vi "fgv_5413_visa.vi"(7 "cmd":T2, 8 "error in":errorcluster) -> (0 "error out":errorcluster)   [LabVIEW 2021]
uses:
  ctrl/PXIe-5413.ctl
  ctrl/rw.ctl
  <instrlib>/niFgen/niFgen.llb/niFgen Output Mode.ctl
  <instrlib>/niFgen/niFgen.llb/niFgen Create Waveform (DBL).vi
panel:
  out "wfm":dbl[](graph)=[0.0, 0.024541228522912288, 0.049067674327418015, 0.07356456359966743, 0.0980171403295606, 0.1224106751992162, 0.14673047445536175, 0.17096188876030122, 0.19509032201612828, 0.2191012401568698, 0.2429801799032639, 0.26671275747489837, 0.2902846772544624, 0.31368174039889146, 0.33688985339222005, 0.3598950365349881, 0.3826834323650898, 0.40524131400498986, 0.4275550934302821, 0.4496113296546066, 0.47139673682599764, 0.49289819222978404, 0.5141027441932218, 0.5349976198870973, 0.5555702330196023, 0.5758081914178453, 0.5956993044924334, 0.6152315905806269, 0.6343932841636455, 0.6531728429537769, 0.6715589548470184, 0.689540544737067, 0.7071067811865476, 0.724247082951467, 0.7409511253549591, 0.7572088465064847, 0.773010453362737, 0.7883464276266063, 0.8032075314806449, 0.8175848131515838, 0.8314696123025452, 0.8448535652497072, 0.8577286100002721, 0.8700869911087116, 0.881921264348355, 0.8932243011955154, 0.9039892931234433, 0.9142097557035308, 0.9238795325112867, 0.9329927988347391, 0.9415440651830208, 0.9495281805930369, 0.9569403357322089, 0.9637760657954401, 0.9700312531945441, 0.9757021300385287, 0.9807852804032305, 0.9852776423889413, 0.989176509964781, 0.9924795345987101, 0.9951847266721969, 0.9972904566786903, 0.9987954562051724, 0.9996988186962044, 1.0, 0.9996988186962044, 0.9987954562051724, 0.9972904566786903, 0.9951847266721969, 0.9924795345987101, 0.989176509964781, 0.9852776423889413, 0.9807852804032305, 0.9757021300385286, 0.9700312531945441, 0.9637760657954398, 0.9569403357322089, 0.9495281805930367, 0.9415440651830208, 0.9329927988347388, 0.9238795325112867, 0.9142097557035306, 0.9039892931234433, 0.8932243011955152, 0.881921264348355, 0.8700869911087113, 0.8577286100002721, 0.844853565249707, 0.8314696123025452, 0.8175848131515836, 0.8032075314806449, 0.7883464276266061, 0.773010453362737, 0.7572088465064843, 0.7409511253549591, 0.7242470829514667, 0.7071067811865476, 0.6895405447370667, 0.6715589548470184, 0.6531728429537765, 0.6343932841636455, 0.6152315905806266, 0.5956993044924334, 0.575808191417845, 0.5555702330196023, 0.5349976198870969, 0.5141027441932218, 0.49289819222978376, 0.4713967368259977, 0.4496113296546063, 0.42755509343028214, 0.4052413140049896, 0.38268343236508984, 0.3598950365349879, 0.3368898533922201, 0.31368174039889124, 0.29028467725446244, 0.26671275747489814, 0.24298017990326395, 0.21910124015686955, 0.19509032201612833, 0.17096188876030097, 0.1467304744553618, 0.12241067519921595, 0.09801714032956065, 0.07356456359966718, 0.04906767432741806, 0.024541228522912045, 3.836381624704177e-17, -0.024541228522912528, -0.04906767432741798, -0.07356456359966766, -0.09801714032956058, -0.12241067519921643, -0.14673047445536172, -0.17096188876030144, -0.19509032201612825, -0.21910124015687, -0.24298017990326387, -0.2667127574748986, -0.29028467725446233, -0.3136817403988917, -0.33688985339222, -0.35989503653498833, -0.3826834323650897, -0.40524131400499, -0.42755509343028203, -0.44961132965460676, -0.4713967368259976, -0.4928981922297842, -0.5141027441932217, -0.5349976198870974, -0.5555702330196022, -0.5758081914178454, -0.5956993044924334, -0.6152315905806269, -0.6343932841636455, -0.6531728429537769, -0.6715589548470184, -0.689540544737067, -0.7071067811865476, -0.724247082951467, -0.7409511253549591, -0.7572088465064846, -0.773010453362737, -0.7883464276266062, -0.8032075314806449, -0.8175848131515836, -0.8314696123025452, -0.844853565249707, -0.8577286100002721, -0.8700869911087113, -0.881921264348355, -0.8932243011955152, -0.9039892931234433, -0.9142097557035306, -0.9238795325112867, -0.9329927988347388, -0.9415440651830208, -0.9495281805930366, -0.9569403357322089, -0.9637760657954397, -0.9700312531945441, -0.9757021300385283, -0.9807852804032305, -0.985277642388941, -0.989176509964781, -0.9924795345987097, -0.9951847266721969, -0.99729045667869, -0.9987954562051724, -0.999698818696204, -1.0, -0.999698818696204, -0.9987954562051724, -0.99729045667869, -0.9951847266721969, -0.9924795345987097, -0.989176509964781, -0.985277642388941, -0.9807852804032305, -0.9757021300385283, -0.9700312531945441, -0.9637760657954396, -0.9569403357322089, -0.9495281805930365, -0.9415440651830208, -0.9329927988347386, -0.9238795325112867, -0.9142097557035304, -0.9039892931234433, -0.893224301195515, -0.881921264348355, -0.8700869911087111, -0.8577286100002721, -0.8448535652497068, -0.8314696123025452, -0.8175848131515834, -0.8032075314806449, -0.7883464276266059, -0.773010453362737, -0.7572088465064842, -0.7409511253549591, -0.7242470829514666, -0.7071067811865476, -0.6895405447370666, -0.6715589548470184, -0.6531728429537764, -0.6343932841636455, -0.6152315905806265, -0.5956993044924334, -0.5758081914178449, -0.5555702330196023, -0.5349976198870968, -0.5141027441932218, -0.49289819222978365, -0.4713967368259977, -0.4496113296546062, -0.42755509343028214, -0.4052413140049895, -0.38268343236508984, -0.3598950365349878, -0.3368898533922201, -0.31368174039889113, -0.29028467725446244, -0.26671275747489803, -0.24298017990326395, -0.21910124015686946, -0.19509032201612833, -0.1709618887603009, -0.1467304744553618, -0.1224106751992159, -0.09801714032956066, -0.07356456359966715, -0.04906767432741807, -0.024541228522912028] caption="Waveform Graph"
  in  "wfm info":T1(array[cluster])=[{"Waveform Type"=0, "Amplitude"=1.0, "# of points"=256}] {"Amplitude" min=0.0 max=1.0 format="%.2f"; "Waveform Type" items=["Sine", "Cosine", "Triangle", "Square", "Sawtooth", "Increasing Ramp", "Decreasing Ramp", "DC Value"]}
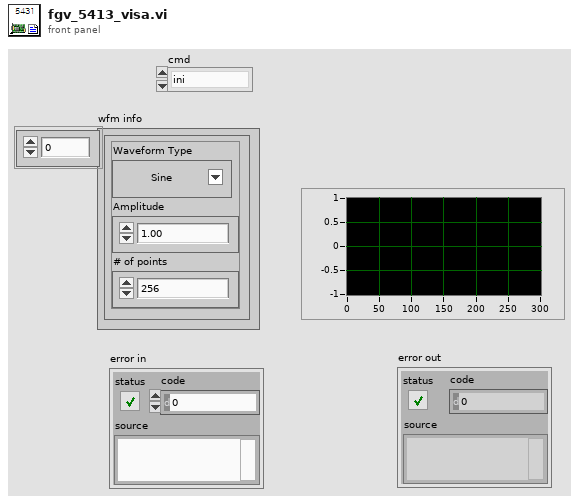
[diagram p1: front panel]
types:
  T1 = cluster{"Waveform Type":u16, "Amplitude":dbl, "# of points":u32}[]
  T2 = typedef "PXIe-5413.ctl" = enum16{"ini", "config", "start", "read", "close"}
  T3 = typedef "rw.ctl" = enum16{"read", "write"}
  T4 = typedef "PXIe-5413_cfg.ctl" = cluster{"visa":refnum<k15>, "DC Offset":dbl, "Digital Filter":bool, "Analog Filter":bool, "Tones":cluster{"Frequency":dbl, "Amplitude":dbl, "Phase":dbl}[], "Sampling Info":cluster{"Frequency":dbl, "Number of Samples":dbl}, "Clock Mode":u32, "Sample Rate (S/s)":dbl, "Gain":dbl, "Sample Clock Source":string}
  T5 = typedef "niFgen Output Mode.ctl" = u32
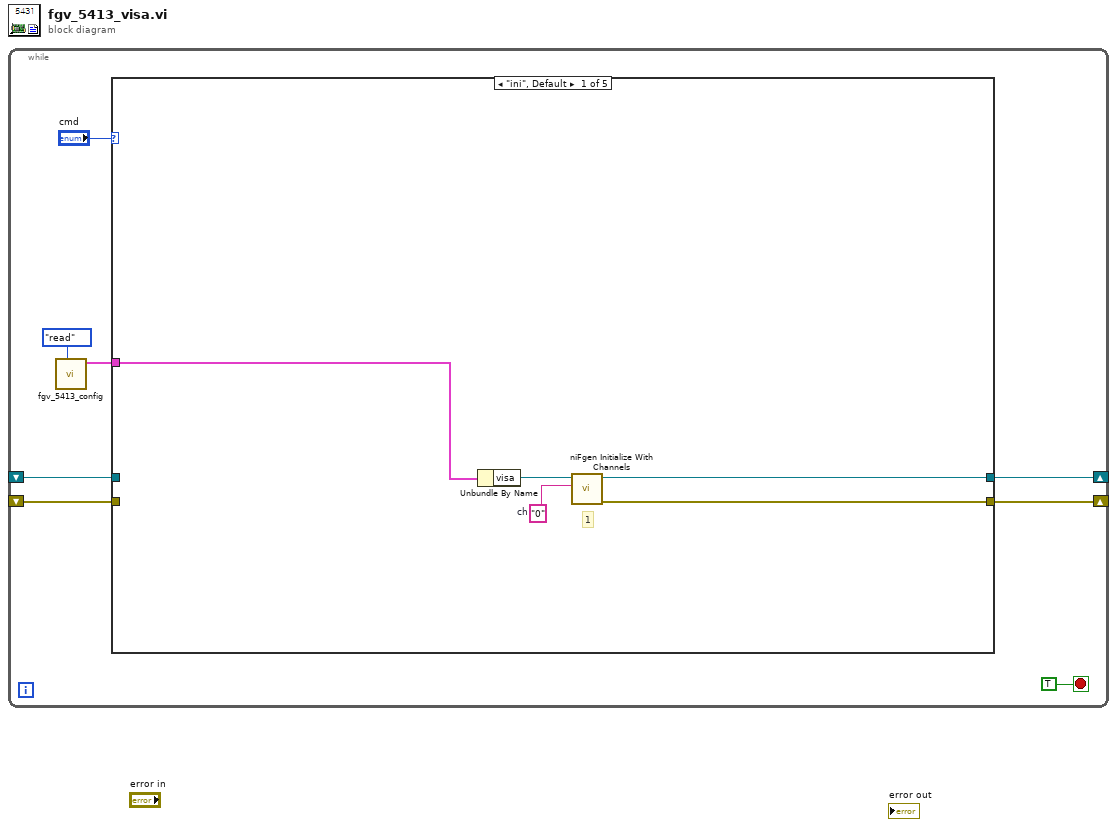
[diagram p0: block diagram]
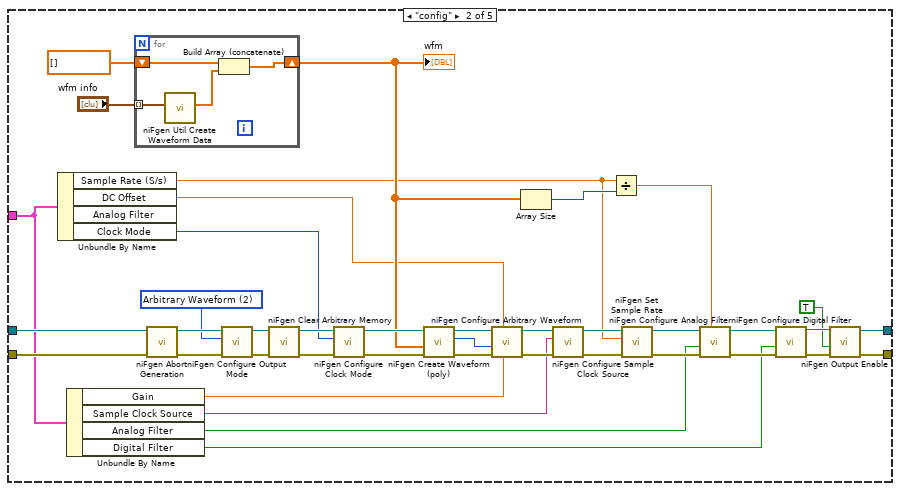
[diagram p2: hidden frame]
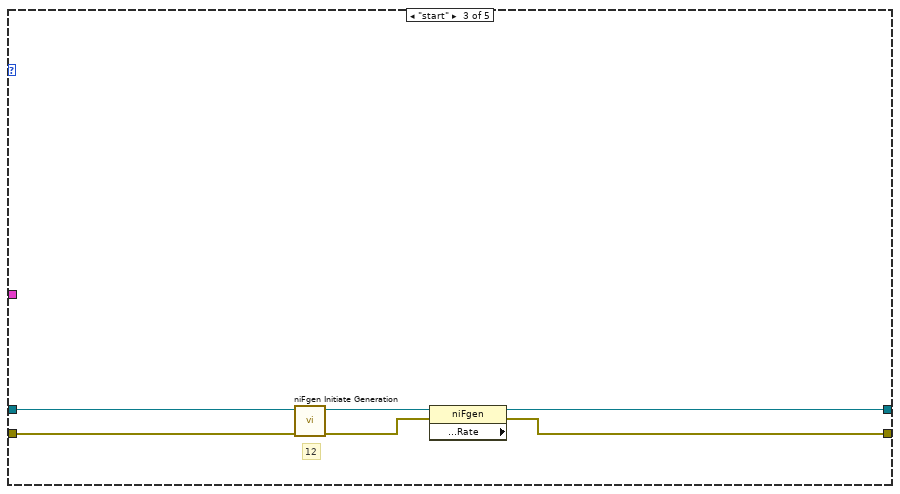
[diagram p3: hidden frame]
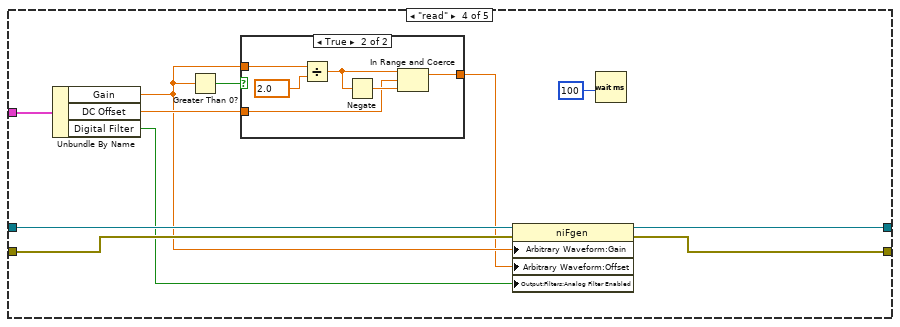
[diagram p4: hidden frame]
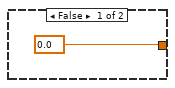
[diagram p5: hidden frame]
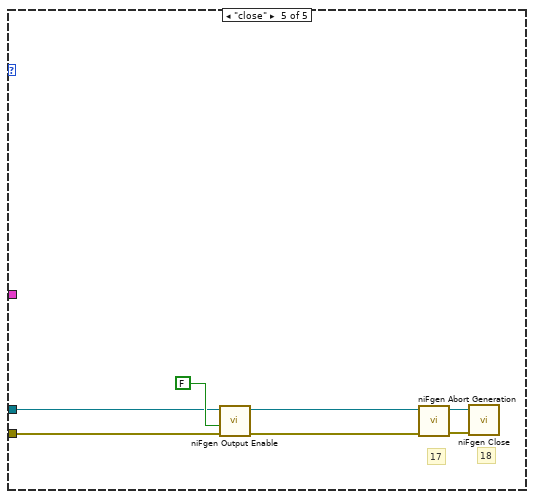
[diagram p6: hidden frame]
diagram:
  n1 = while {
    shift-right: [w6] -> _
    shift-left: _ -> [w4]
    shift-right: [w5] -> _
    shift-left: _ -> [w3]
    stop <- TRUE stop-if-true
    n2 = call "fgv_5413_config.vi"("cmd"=rw."read") -> ("config 2"=w1:T4)  [unwired: 10 in]
    n3 = case shown="\"ini\", Default" "cmd" {
      tunnel: [w11 w40 w59 w72 _] -> w6
      tunnel: [w10 w41 w58 w71 _] -> w5
      tunnel: w4 -> [_ w39 w63 w73 w85]
      tunnel: w3 -> [_ w38 w62 w74 w84]
      tunnel: w1 -> [w9 w20 _ w68 _]
      frame "ini", Default {
        w13 = "0"  # ch
        # "1"
        n4 = Unbundle By Name(w9) -> ("visa"=w12:refnum<k15>)
        n5 = call <instrlib>:"niFgen Initialize With Channels.vi"("Channel Name"=w13, "Resource Name"=w12) -> ("error out"=w10:errorcluster, "Instrument Handle Out"=w11:refnum<k15>)  [unwired: 8 in]
      }
      frame "config" {
        w49 = T5 2 items=["Standard Function", "Frequency List", "Arbitrary Waveform", "Arbitrary Sequence", "Script"] ("Output Mode")
        n6 = Unbundle By Name(w20) -> ("Sample Rate (S/s)"=w23:dbl, "DC Offset"=w14:dbl, "Clock Mode"=w21:u32)  [unwired: 1 out]
        n7 = Unbundle By Name(w20) -> ("Gain"=w18:dbl, "Sample Clock Source"=w17:string, "Analog Filter"=w16:bool, "Digital Filter"=w15:bool)
        n8 = for {
          shift-right: [w54] -> w24
          shift-left: dbl[] [] -> [w57]
          tunnel: "wfm info" -> [w55] mode=indexing
          n9 = call <instrlib>:"niFgen Util Create Waveform Data.vi"("Waveform"=w55) -> ("Waveform Data"=w56:dbl[])  [unwired: 10 in]
          n10 = Build Array (concatenate)(w57, w56) -> (w54:dbl[])
        }
        "wfm" <- w24
        n11 = call <instrlib>:"niFgen Abort Generation.vi"("error in (no error)"=w38, "Instrument Handle"=w39) -> ("error out"=w37:errorcluster, "Instrument Handle Out"=w52:refnum<k15>)  [unwired: 8 in]
        n12 = call <instrlib>:"niFgen Configure Output Mode.vi"("error in (no error)"=w37, "Output Mode (default: 0=Standard Function)"=w49, "Instrument Handle"=w52) -> ("error out"=w36:errorcluster, "Instrument Handle Out"=w48:refnum<k15>)  [unwired: 6 in]
        n13 = call <instrlib>:"niFgen Clear Arbitrary Memory.vi"("error in (no error)"=w36, "Instrument Handle"=w48) -> ("error out"=w35:errorcluster, "Instrument Handle Out"=w47:refnum<k15>)  [unwired: 8 in]
        n14 = call <instrlib>:"niFgen Configure Clock Mode.vi"("error in (no error)"=w35, "Clock Mode (default: 1=divide down)"=w21, "Instrument Handle"=w47) -> ("error out"=w34:errorcluster, "Instrument Handle Out"=w51:refnum<k15>)  [unwired: 7 in]
        n15 = call-poly <instrlib>:"niFgen Create Waveform (poly).vi"("error in (no error)"=w34, "Waveform Data Array"=w24, "Instrument Handle"=w51) -> ("error out"=w33:errorcluster, "Waveform Handle"=w19:i32, "Instrument Handle Out"=w53:refnum<k15>)  [unwired: 6 in]
        n16 = call <instrlib>:"niFgen Configure Arbitrary Waveform.vi"("Gain"=w18, "Offset"=w14, "error in (no error)"=w33, "Waveform Handle"=w19, "Instrument Handle"=w53) -> ("error out"=w32:errorcluster, "Instrument Handle Out"=w50:refnum<k15>)  [unwired: 5 in]
        n17 = Array Size(array=w24) -> (size(s)=w25:i32)
        n18 = call <instrlib>:"niFgen Configure Sample Clock Source.vi"("error in (no error)"=w32, "Source (Onboard Clock)"=w17, "Instrument Handle"=w50) -> ("error out"=w31:errorcluster, "Instrument Handle Out"=w46:refnum<k15>)  [unwired: 7 in]
        n19 = Divide(x=w23, y=w25) -> (x/y=w22:dbl)
        n20 = call <instrlib>:"niFgen Set Sample Rate.vi"("error in (no error)"=w31, "Sample Rate (Samp/s)"=w23, "Instrument Handle"=w46) -> ("error out"=w30:errorcluster, "Instrument Handle Out"=w45:refnum<k15>)  [unwired: 7 in]
        n21 = call <instrlib>:"niFgen Configure Analog Filter.vi"("Filter Correction Frequency"=w22, "error in (no error)"=w30, "Analog Filter Enable (default: True)"=w16, "Instrument Handle"=w45) -> ("error out"=w29:errorcluster, "Instrument Handle Out"=w44:refnum<k15>)  [unwired: 6 in]
        n22 = call <instrlib>:"niFgen Configure Digital Filter.vi"("error in (no error)"=w29, "Digital Filter Enable (default: True)"=w15, "Instrument Handle"=w44) -> ("error out"=w28:errorcluster, "Instrument Handle Out"=w43:refnum<k15>)  [unwired: 7 in]
        n23 = call <instrlib>:"niFgen Output Enable.vi"("error in (no error)"=w28, "Output Enable (default: True)"=TRUE ("output enable"), "Instrument Handle"=w43) -> ("error out"=w41:errorcluster, "Instrument Handle Out"=w40:refnum<k15>)  [unwired: 7 in]
      }
      frame "start" {
        # "12"
        n24 = call <instrlib>:"niFgen Initiate Generation.vi"("error in (no error)"=w62, "Instrument Handle"=w63) -> ("error out"=w60:errorcluster, "Instrument Handle Out"=w61:refnum<k15>)  [unwired: 8 in]
        n25 = property class="niFgen" props=["Clocks:Sample Clock:Rate"](reference=w61, error in=w60) -> (reference out=w59:refnum<k15>, error out=w58:errorcluster)  [unwired: 1 out]
      }
      frame "read" {
        n26 = Unbundle By Name(w68) -> ("Gain"=w66:dbl, "DC Offset"=w67:dbl, "Digital Filter"=w64:bool)
        n27 = Greater Than 0?(x=w66) -> (x > 0?=w69:bool)
        n28 = case shown="True" w69 {
          tunnel: w66 -> [_ w80]
          tunnel: [0.0 ("DC Offset") w76] -> w65
          tunnel: w67 -> [_ w77]
          frame False {
          }
          frame True {
            n29 = Divide(x=w80, y=2.0) -> (x/y=w79:dbl)
            n30 = Negate(x=w79) -> (-x=w78:dbl)
            n31 = In Range and Coerce(upper limit=w79, x=w77, lower limit=w78) -> (coerced(x)=w76:dbl)  [unwired: 1 out]
          }
        }
        n32 = property class="niFgen"(reference=w73, error in=w74, "Arbitrary Waveform:Gain"=w66, "Arbitrary Waveform:Offset"=w65, "Output:Filters:Analog Filter Enabled"=w64) -> (reference out=w72:refnum<k15>, error out=w71:errorcluster)
        n33 = Wait (ms)(milliseconds to wait=u32 100 ("millisecond multiple")) -> ()  [unwired: 1 out]
      }
      frame "close" {
        # "18"
        # "17"
        n34 = call <instrlib>:"niFgen Output Enable.vi"("error in (no error)"=w84, "Output Enable (default: True)"=FALSE ("output enable"), "Instrument Handle"=w85) -> ("error out"=w82:errorcluster, "Instrument Handle Out"=w83:refnum<k15>)  [unwired: 7 in]
        n35 = call <instrlib>:"niFgen Abort Generation.vi"("error in (no error)"=w82, "Instrument Handle"=w83) -> ("error out"=w88:errorcluster, "Instrument Handle Out"=w87:refnum<k15>)  [unwired: 8 in]
        n36 = call <instrlib>:"niFgen Close.vi"("error in (no error)"=w88, "Instrument Handle"=w87) -> ()  [unwired: 9 in, 1 out]
      }
    }
  }
